vi "create.vi"(5 "subprotocols":string[](array[string]), 7 "host header":string, 8 "error in":errorcluster, 9 "url":string, 10 "port":u16=80, 11 "address":string) -> (0 "error out":errorcluster, 3 "websocket client out":refnum<class "websocket client.lvclass">)   [LabVIEW 2016, in "websocket client.lvclass"]
uses:
  websocket client.lvclass
  websocket client.lvclass/websocket client.ctl
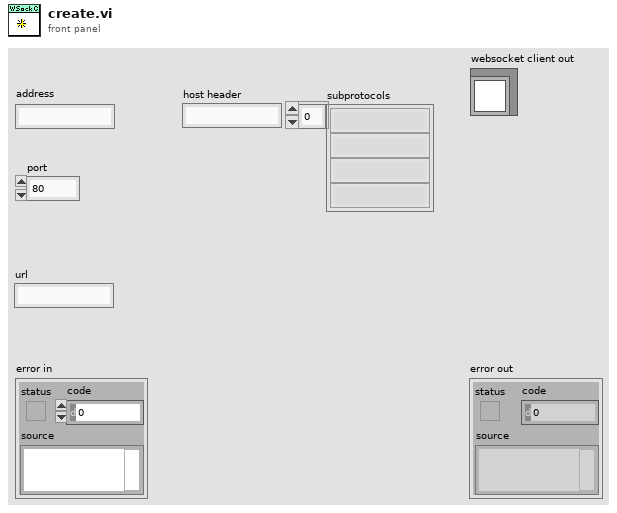
[diagram p1: front panel]
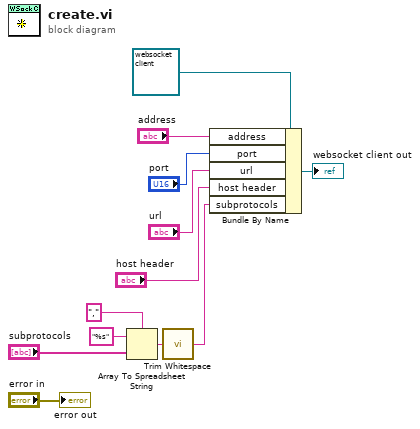
[diagram p0: block diagram]
diagram:
  n1 = Array To Spreadsheet String(delimiter (Tab)=",", array="subprotocols", 3:"%s" ("format string")) -> (spreadsheet string=w2:string)
  n2 = call <vilib>:"Trim Whitespace.vi"("string"=w2) -> ("trimmed string"=w1:string)  [unwired: 1 in]
  n3 = Bundle By Name(cluster=refnum<class "websocket client.lvclass"> refnum ("websocket client out"), "address"="address", "port"="port", "url"="url", "host header"="host header", "subprotocols"=w1) -> (→"websocket client out":refnum<class "websocket client.lvclass">)
  "error out" <- "error in"
